vi "pack tcp packet.vi"(7 "tcp-message-type":T1=enum."cmd", 11 "String":string) -> (3 "TCP Pack":string)   [LabVIEW 2020, in "CSM-TCP-Router.lvlib"]
uses:
  CSM-TCP-Router.lvlib
  tcp-msg type.ctl
  <userlib>/_NEVSTOP/Communicable State Machine(CSM)/addons/MassData-Parameter/_support/Operation-FGV-MassData.ctl
  <userlib>/_NEVSTOP/Communicable State Machine(CSM)/addons/MassData-Parameter/CSM MassData Parameter Support.lvlib
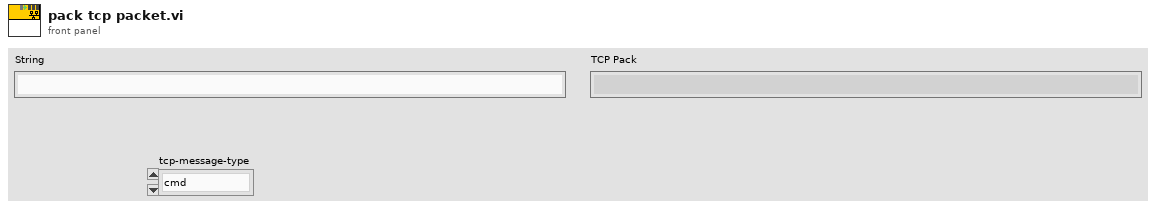
[diagram p1: front panel]
types:
  T1 = typedef "CSM-TCP-Router.lvlib/tcp-msg type.ctl" = enum8{"info", "error", "cmd", "cmd-resp", "resp", "async-resp", "status", "interrupt"}
  T2 = typedef "CSM MassData Parameter Support.lvlib/Operation-FGV-MassData.ctl" = enum16{"Initialize", "Read", "Write", "Status", "Release"}
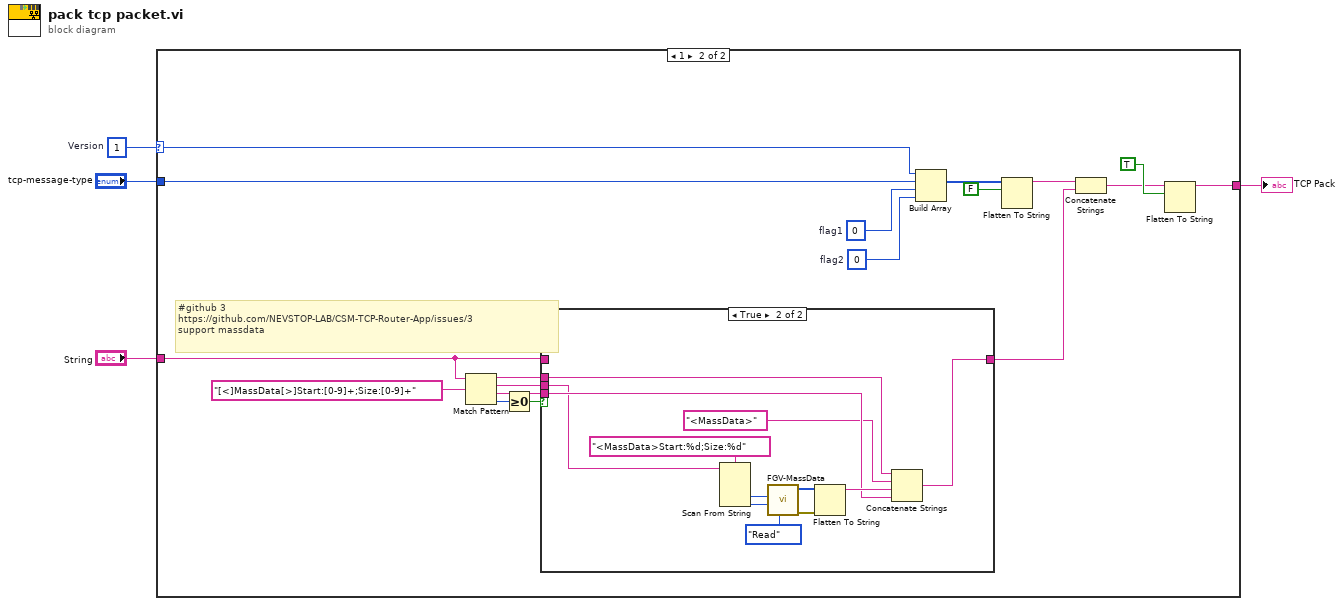
[diagram p0: block diagram]
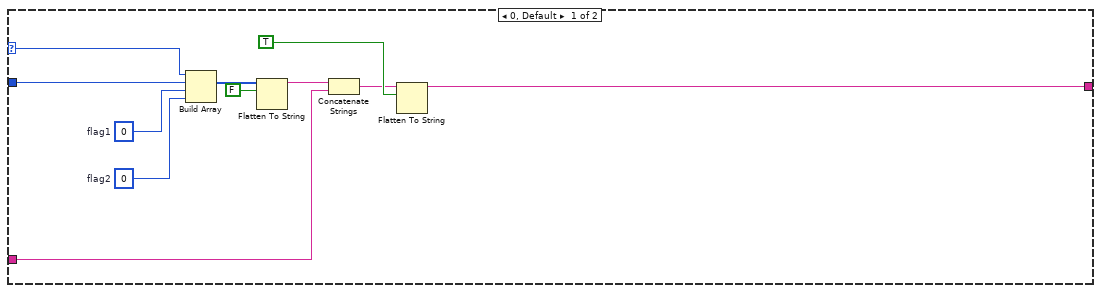
[diagram p2: hidden frame]
diagram:
  w1 = u8 1  # Version
  n1 = case shown="1" w1 {
    selector: w1 -> [w5 w24]
    tunnel: "String" -> [w14 w17]
    tunnel: [w13 w32] -> w3
    tunnel: "tcp-message-type" -> [w11 w30]
    frame 0, Default {
      w6 = u8 0  # flag2
      w7 = u8 0  # flag1
      n2 = Build Array(w5, w11, w7, w6) -> (w8:u8[])
      n3 = Flatten To String(anything=w8, prepend array or string size? (T)=FALSE) -> (data string=w9:string)  [unwired: 1 in, 3 out]
      n4 = Concatenate Strings(w9, w14) -> (w12:string)
      n5 = Flatten To String(anything=w12, prepend array or string size? (T)=TRUE) -> (data string=w13:string)  [unwired: 1 in, 3 out]
    }
    frame 1 {
      w25 = u8 0  # flag2
      w26 = u8 0  # flag1
      # "#github 3\nhttps://github.com/NEVSTOP-LAB/CSM-TCP-Router-App/issues/3\nsupport massdata"
      n6 = Match Pattern(string=w17, regular expression="[<]MassData[>]Start:[0-9]+;Size:[0-9]+" ("string")) -> (before substring=w22:string, match substring=w20:string, after substring=w21:string, offset past match=w19:i32)  [unwired: 1 in]
      n7 = Greater Or Equal To 0?(x=w19) -> (x >= 0?=w18:bool)
      n8 = case shown="True" w18 {
        tunnel: w22 -> [_ w41]
        tunnel: w21 -> [_ w40]
        tunnel: [w34 w39] -> w16
        tunnel: w20 -> [_ w38]
        tunnel: w17 -> [w34 _]
        frame False {
        }
        frame True {
          n9 = Scan From String(format string="<MassData>Start:%d;Size:%d", input string=w38) -> (output 1=w45:i32, output 2=w44:i32)  [unwired: 4 in, 3 out]
          n10 = call <userlib>:"FGV-MassData.vi"("Operation"=Operation-FGV-MassData."Read", "size"=w44, "Start"=w45) -> ("Error out"=w35:errorcluster, "Data out"=w43:u8[])  [unwired: 5 in, 2 out]
          n11 = Flatten To String(anything=w43, error in (no error)=w35) -> (data string=w42:string)  [unwired: 2 in, 2 out]
          n12 = Concatenate Strings(w41, "<MassData>" ("format string"), w42, w40) -> (w39:string)
        }
      }
      n13 = Build Array(w24, w30, w26, w25) -> (w27:u8[])
      n14 = Flatten To String(anything=w27, prepend array or string size? (T)=FALSE) -> (data string=w28:string)  [unwired: 1 in, 3 out]
      n15 = Concatenate Strings(w28, w16) -> (w31:string)
      n16 = Flatten To String(anything=w31, prepend array or string size? (T)=TRUE) -> (data string=w32:string)  [unwired: 1 in, 3 out]
    }
  }
  "TCP Pack" <- w3
